vi "Data Channel.vi"(8 "error in (no error)":errorcluster, 11 "Node Ptr":T6 format="%.0x") -> (0 "error out":errorcluster)   [LabVIEW 2018, in "Instrument Addon System Explorer.lvlib"]
uses:
  Instrument Addon System Explorer.lvlib
  <vilib>/NI Veristand/Custom Device API/Custom Device Item Ref.ctl
  Addon Shared/Types/Protocol Data Type.ctl
  Addon Shared/Types/Data Channel Type.ctl
  Addon Shared/Types/Type Cast Type.ctl
  Addon Shared/Types/Endian.ctl
  Addon Shared/Types/FG Control.ctl
  <vilib>/NI Veristand/Custom Device API/Custom Device Channel.ctl
  <vilib>/NI Veristand/Custom Device API/Custom Device Channel Type.ctl
  Addon Shared/SubVIs/Constants.vi
  <vilib>/NI Veristand/Custom Device API/NI VeriStand - Get Item Property.vi
  <vilib>/NI Veristand/Custom Device API/Get Item Property (U32).vi
  <vilib>/NI Veristand/Custom Device API/Get Item Property (String).vi
  <vilib>/NI Veristand/Custom Device API/Get Item Property (String Array).vi
  <vilib>/NI Veristand/Custom Device API/NI VeriStand - Set Item Property.vi
  <vilib>/NI Veristand/Custom Device API/Set Item Property (U32).vi
  <vilib>/NI Veristand/Custom Device API/Set Item Property (String).vi
  <vilib>/NI Veristand/Custom Device API/Set Item Property (String Array).vi
  <vilib>/NI Veristand/Custom Device API/NI VeriStand - Set Custom Device Channel Value Table.vi
  <vilib>/NI Veristand/Custom Device API/Custom Device API.lvlib
  Addon Shared/Instrument Addon Shared.lvlib
panel:
  in  "Delimiter":string=","
  in  "Reset":bool
  in  "Create":bool
  in  "Elements":u32
  in  "Units":string
  in  "Default Value":dbl
  in  "SHDocVw.IWebBrowser":refnum<k7>(container)
  out "Channel Type (Tab)":T1(tab)
  in  "Test Value":dbl
  in  "Format String":string="%.3g"
  out "Validated String":string
  in  "Expected String":string caption="Expected String (case sensitive)"
  in  "Endian":T2=enum."Little"
  in  "Type":T3
  in  "Enumerated List":i32(listbox)
  in  "Add":bool
  in  "Remove":bool
  in  "Channel Type":T4
  out "Data Type":T5
  in  "Header":cluster{"Section Name":string}={"Section Name"="Data Settings"}
  in  "Description":string
  in  "Name":string
  in  "Header 2":cluster{"Section Name":string}={"Section Name"="Data Format Settings"}
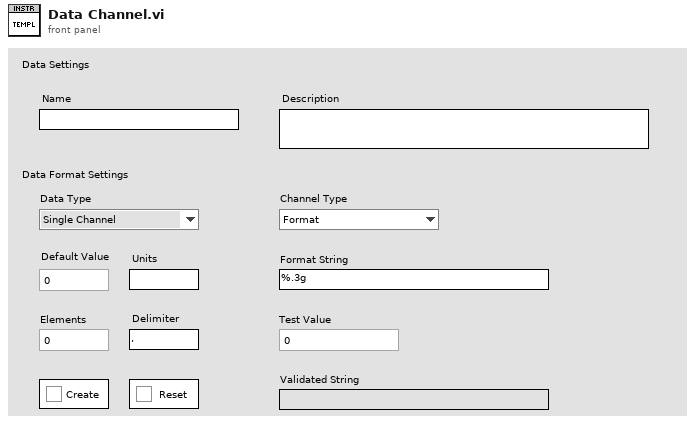
[diagram p1: front panel]
types:
  T1 = enum32{"Format", "Comparison", "Type Cast", "List"}
  T2 = typedef "Instrument Addon Shared.lvlib/Endian.ctl" = enum16{"Native", "Little", "Big"}
  T3 = typedef "Instrument Addon Shared.lvlib/Type Cast Type.ctl" = enum16{"DBL", "SGL", "U64", "U32", "U16", "U8", "I64", "I32", "I16", "I8"}
  T4 = typedef "Instrument Addon Shared.lvlib/Data Channel Type.ctl" = enum16{"Format", "Comparison", "Type Cast", "Enumerated List"}
  T5 = typedef "Instrument Addon Shared.lvlib/Protocol Data Type.ctl" = enum16{"Single Channel", "Array"}
  T6 = typedef "Custom Device API.lvlib/Custom Device Item Ref.ctl" = u64
  T7 = typedef "Instrument Addon Shared.lvlib/FG Control.ctl" = enum16{"Get", "Set"}
  T8 = typedef "Custom Device API.lvlib/Custom Device Item Info.ctl" = cluster{"Name":string, "Is Channel":bool, "GUID":string, "Is Waveform":bool}
  T9 = typedef "Instrument Addon Shared.lvlib/Data Parameters.ctl" = cluster{"Data Type":T5, "Channel Type":T4, "Format String":string, "Expected String":string, "Type":T3, "List":string[], "Delimiter":string, "Endian":T2}
  T10 = typedef "Custom Device API.lvlib/Custom Device Channel.ctl" = cluster{"Type":T11, "Units":string, "Default Value":dbl, "Faultable":bool, "Scalable":bool}
  T11 = typedef "Custom Device API.lvlib/Custom Device Channel Type.ctl" = enum16{"Input", "Output"}
  T12 = typedef "Custom Device API.lvlib/Custom Device Commands.ctl" = enum16{"Default", "Item renamed", "Shutdown", "Dynamic button pressed"}
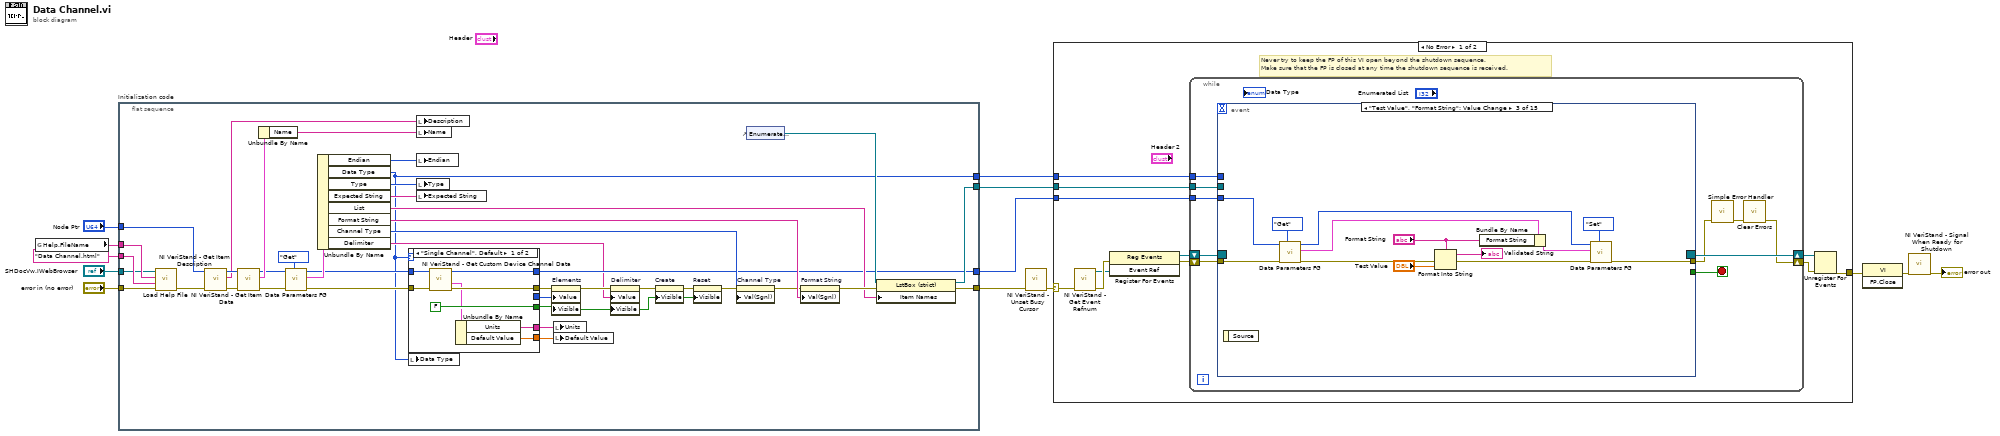
[diagram p0: block diagram]
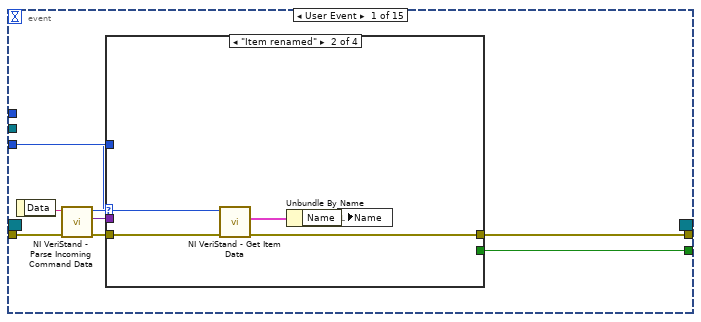
[diagram p2: hidden frame]
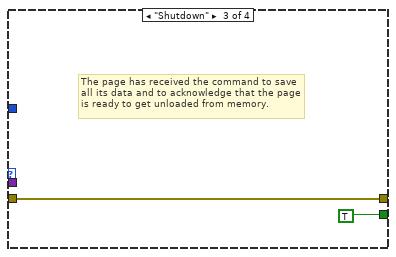
[diagram p4: hidden frame]
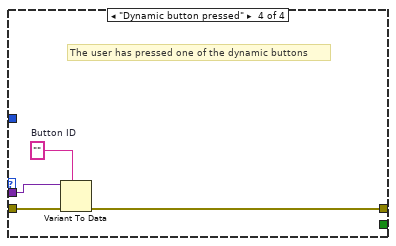
[diagram p5: hidden frame]
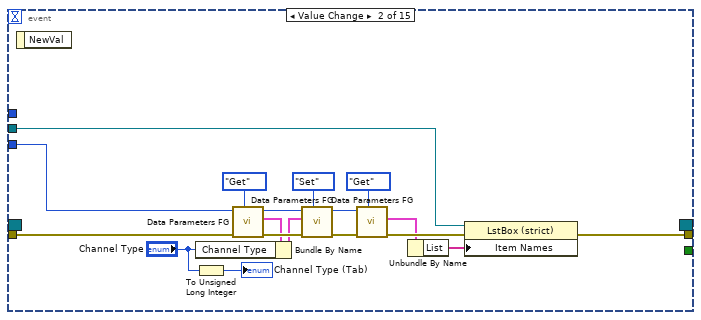
[diagram p6: hidden frame]
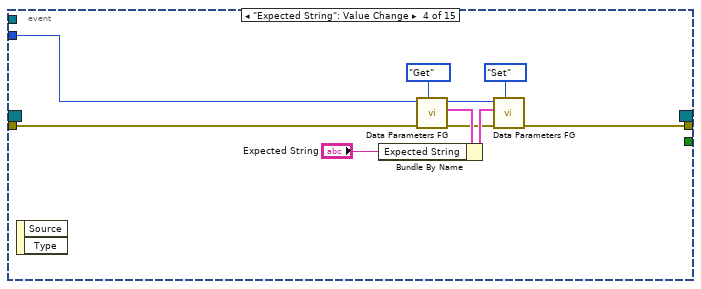
[diagram p7: hidden frame]
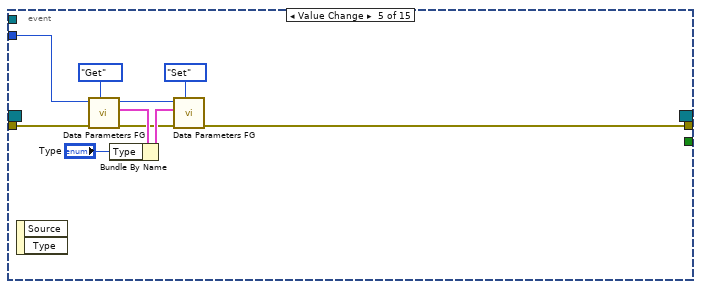
[diagram p8: hidden frame]
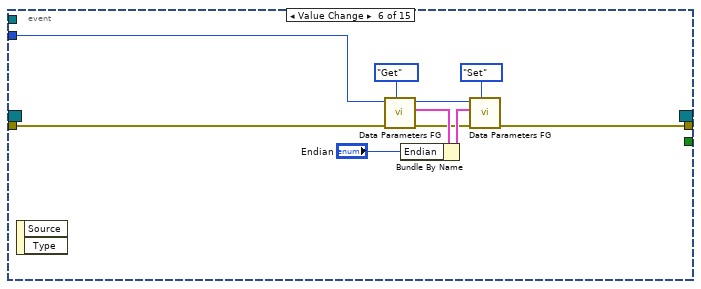
[diagram p9: hidden frame]
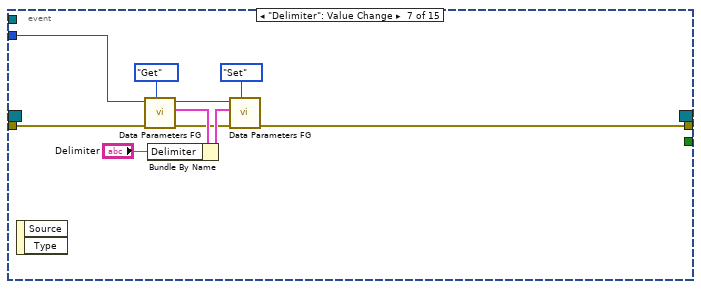
[diagram p10: hidden frame]
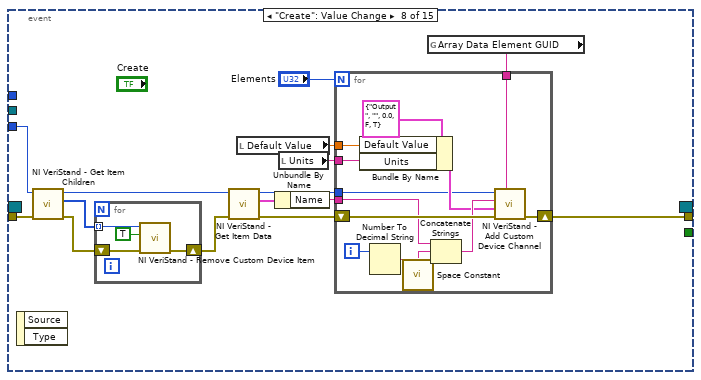
[diagram p11: hidden frame]
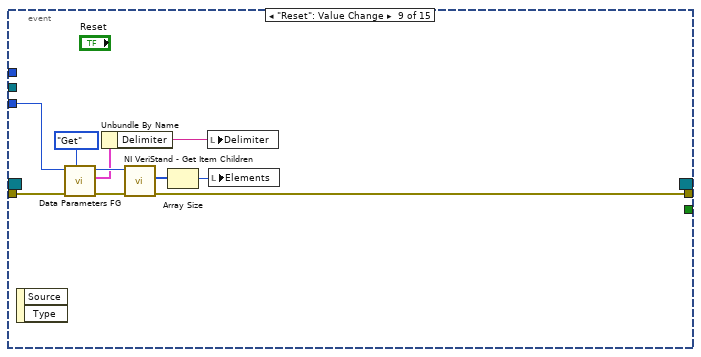
[diagram p12: hidden frame]
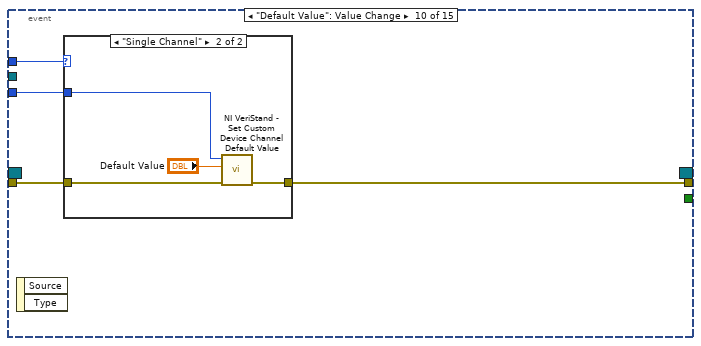
[diagram p13: hidden frame]
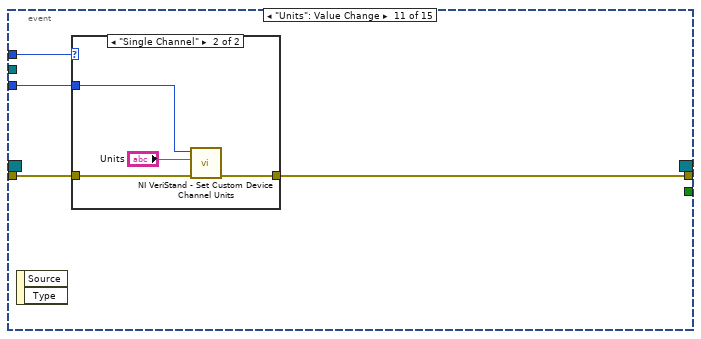
[diagram p15: hidden frame]
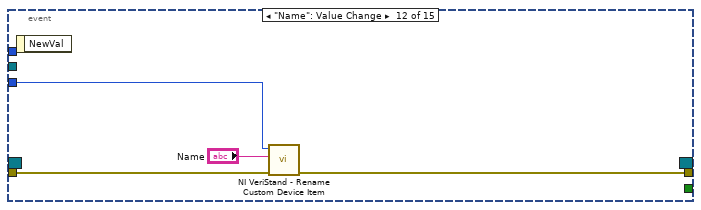
[diagram p17: hidden frame]
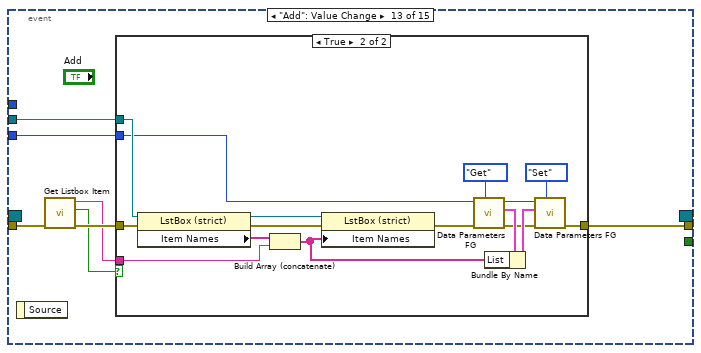
[diagram p18: hidden frame]
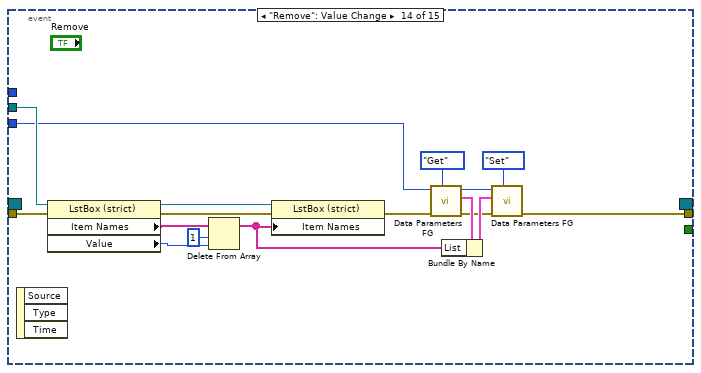
[diagram p20: hidden frame]
diagram:
  n1 = global read "Constants.vi" "Help.FileName"() -> (w1:string)
  n2 = flat-sequence "Initialization code" {
    tunnel: "error in (no error)" -> [w47]
    tunnel: "Node Ptr" -> [w52]
    tunnel: [w34] -> w9
    tunnel: [w26] -> w6
    tunnel: w1 -> [w45]
    tunnel: "Data Channel.html" ("HTML File") -> [w44]
    tunnel: "SHDocVw.IWebBrowser" -> [w43]
    tunnel: [w31] -> w3
    tunnel: [w16] -> w2
    frame #0 {
      n3 = call "Load Help File.vi"("error in (no error)"=w47, "HTML File"=w44, "Main CHM File"=w45, "SHDocVw.IWebBrowser2"=w43) -> ("error out"=w46:errorcluster)  [unwired: 7 in]
      n4 = call <vilib>:"NI VeriStand - Get Item Description.vi"("error in (no error)"=w46, "Item Ref in"=w52) -> ("error out"=w50:errorcluster, "Description"=w51:string, "Item Ref out"=w53:T6)  [unwired: 7 out]
      n5 = call <vilib>:"NI VeriStand - Get Item Data.vi"("error in (no error)"=w50, "Item Ref in"=w53) -> ("error out"=w30:errorcluster, "Item Info"=w49:T8, "Item Ref out"=w29:T6)  [unwired: 7 out]
      n6 = Unbundle By Name(w49) -> ("Name"=w48:string)
      n7 = call "Data Parameters FG.vi"("Action"=FG_Control."Get", "error in (no error)"=w30, "Item Ref in"=w29) -> ("error out"=w28:errorcluster, "Data Parameters"=w41:T9, "Item Ref out"=w27:T6)  [unwired: 6 in]
      n8 = Unbundle By Name(w41) -> ("Endian"=w15:T2, "Data Type"=w16:T5, "Type"=w36:T3, "Expected String"=w37:string, "List"=w32:string[], "Format String"=w40:string, "Channel Type"=w39:T4, "Delimiter"=w17:string)
      n9 = case shown="\"Single Channel\", Default" w16 {
        tunnel: [FALSE TRUE] -> w14
        tunnel: w28 -> [w60 w65]
        tunnel: w27 -> [w59 w69]
        tunnel: [w58 w64] -> w19
        tunnel: [w57 w66] -> w26
        tunnel: [w55 ""] -> w25
        tunnel: [w54 0.0 ("Default Value")] -> w24
        tunnel: [_ w62] -> w18
        frame "Single Channel", Default {
          n10 = call <vilib>:"NI VeriStand - Get Custom Device Channel Data.vi"("error in (no error)"=w60, "Channel Ref in"=w59) -> ("error out"=w58:errorcluster, "Channel"=w56:T10, "Channel Ref out"=w57:T6)  [unwired: 4 in, 3 out]
          n11 = Unbundle By Name(w56) -> ("Units"=w55:string, "Default Value"=w54:dbl)
        }
        frame "Array" {
          n12 = call <vilib>:"NI VeriStand - Get Item Children.vi"("error in (no error)"=w65, "Item Ref in"=w69) -> ("error out"=w64:errorcluster, "Child Refs"=w63:T6[], "Item Ref out"=w66:T6)  [unwired: 6 in, 1 out]
          n13 = Array Size(array=w63) -> (size(s)=w62:i32)
        }
      }
      n14 = local write "Data Type"(w16) -> ()
      n15 = local write "Description"(w51) -> ()
      n16 = local write "Name"(w48) -> ()
      n17 = local write "Endian"(w15) -> ()
      n18 = local write "Type"(w36) -> ()
      n19 = local write "Expected String"(w37) -> ()
      n20 = property on="Elements" class="DigNum (strict)"(error in=w19, "Value"=w18, "Visible"=w14) -> (error out=w23:errorcluster)  [unwired: 1 in, 1 out]
      n21 = local write "Units"(w25) -> ()
      n22 = local write "Default Value"(w24) -> ()
      n23 = property on="Delimiter" class="Str"(error in=w23, "Value"=w17, "Visible"=w14) -> (error out=w22:errorcluster)  [unwired: 1 in, 1 out]
      n24 = property on="Create" class="Bool"(error in=w22, "Visible"=w14) -> (error out=w21:errorcluster)  [unwired: 1 in, 1 out]
      n25 = property on="Reset" class="Bool"(error in=w21, "Visible"=w14) -> (error out=w20:errorcluster)  [unwired: 1 in, 1 out]
      n26 = property on="Channel Type" class="Enum (strict)"(error in=w20, "Val(Sgnl)"=w39) -> (error out=w38:errorcluster)  [unwired: 1 in, 1 out]
      n27 = control-ref of="Enumerated List"() -> (w33:refnum<vi>)
      n28 = property on="Format String" class="Str"(error in=w38, "Val(Sgnl)"=w40) -> (error out=w35:errorcluster)  [unwired: 1 in, 1 out]
      n29 = property class="LstBox (strict)"(reference=w33, error in=w35, "Item Names"=w32) -> (reference out=w31:refnum<vi>, error out=w34:errorcluster)
    }
  }
  n30 = call <vilib>:"NI VeriStand - Unset Busy Cursor.vi"("error in (no error)"=w9) -> ("error out"=w8:errorcluster)  [unwired: 10 out]
  n31 = case shown="No Error" w8 {
    selector: w8 -> [w73 w294]
    tunnel: [w78 w292] -> w13
    tunnel: w6 -> [w74 _]
    tunnel: w3 -> [w72 _]
    tunnel: w2 -> [w71 _]
    frame No Error {
      # "Never try to keep the FP of this VI open beyond the shutdown sequence.\nMake sure that the FP is closed at any time the shutdown sequence is received."
      n32 = call <vilib>:"NI VeriStand - Get Event Refnum.vi"("error in (no error)"=w73) -> ("error out"=w81:errorcluster, "Event Ref"=w77:refnum<user-event>)  [unwired: 9 out]
      n33 = register-events(error in=w81, w77) -> (reference out=w75:refnum<event-registration>, error out=w76:errorcluster)  [unwired: 1 in]
      n34 = while {
        tunnel: w74 -> [w87]
        shift-right: [w84] -> w79
        shift-left: w76 -> [w90]
        shift-right: [w91] -> w80
        shift-left: w75 -> [w89]
        tunnel: w72 -> [w83]
        tunnel: w71 -> [w82]
        stop <- w88 stop-if-true
        n35 = event shown="[2] \"Test Value\", \"Format String\": Value Change" {
          selector: w89 -> [_ _ _ _ _ _ _ _ _ _ _ _ _ _ _]
          dyn-events: [_ _ _ _ _ _ _ _ _ _ _ _ _ _ _] -> w91
          timeout: _ -> [_ _ _ _ _ _ _ _ _ _ _ _ _ _ _]
          tunnel: w90 -> [w99 w123 w140 w150 w160 w170 w180 w184 w222 w228 w237 w246 w248 w273 w290]
          tunnel: [w95 _ _ _ _ _ _ _ _ _ _ _ _ _ _] -> w88
          tunnel: [w94 w112 w139 w149 w153 w169 w179 w186 w215 w227 w236 w245 w247 w274 w289] -> w86
          tunnel: w87 -> [w93 w121 w138 w148 w159 w168 w178 w183 w220 w226 w235 w244 w250 w271 w291]
          tunnel: w83 -> [_ w114 _ _ _ _ _ _ _ _ _ _ w249 w272 _]
          tunnel: w82 -> [_ _ _ _ _ _ _ _ _ w225 w234 _ _ _ _]
          event User Event {
            n36 = event-data() -> ("Data"=w98:string)  [unwired: 1 out]
            n37 = call <vilib>:"NI VeriStand - Parse Incoming Command Data.vi"("error in (no error)"=w99, "Incoming data"=w98) -> ("error out"=w97:errorcluster, "Outgoing data"=w92:variant, "Action"=w96:T12)  [unwired: 7 out]
            n38 = case shown="\"Item renamed\"" w96 {
              tunnel: w97 -> [w100 w105 w106 w111]
              tunnel: [_ _ TRUE _] -> w95
              tunnel: [w100 w102 w106 w108] -> w94
              tunnel: w93 -> [_ w104 _ _]
              tunnel: w92 -> [_ _ _ w110]
              frame "Default", Default {
              }
              frame "Item renamed" {
                n39 = call <vilib>:"NI VeriStand - Get Item Data.vi"("error in (no error)"=w105, "Item Ref in"=w104) -> ("error out"=w102:errorcluster, "Item Info"=w103:T8)  [unwired: 8 out]
                n40 = Unbundle By Name(w103) -> ("Name"=w101:string)
                n41 = local write "Name"(w101) -> ()
              }
              frame "Shutdown" {
                # "The page has received the command to save all its data and to acknowledge that the page is ready to get unloaded from memory."
              }
              frame "Dynamic button pressed" {
                w109 = ""  # Button ID
                # "The user has pressed one of the dynamic buttons"
                n42 = Variant To Data(error in=w111, type=w109, Variant=w110) -> (error out=w108:errorcluster)  [unwired: 1 out]
              }
            }
          }
          event Value Change {
            n43 = event-data() -> ()  [unwired: 2 out]
            n44 = To Unsigned Long Integer(number="Channel Type") -> (unsigned 32bit integer=→"Channel Type (Tab)":u32)
            n45 = call "Data Parameters FG.vi"("Action"=FG_Control."Get", "error in (no error)"=w123, "Item Ref in"=w121) -> ("error out"=w129:errorcluster, "Data Parameters"=w125:T9, "Item Ref out"=w127:T6)  [unwired: 6 in]
            n46 = Bundle By Name(cluster=w125, "Channel Type"="Channel Type") -> (w126:T9)
            n47 = call "Data Parameters FG.vi"("Action"=FG_Control."Set", "error in (no error)"=w129, "Data Parameters"=w126, "Item Ref in"=w127) -> ("error out"=w116:errorcluster, "Item Ref out"=w115:T6)  [unwired: 5 in, 1 out]
            n48 = call "Data Parameters FG.vi"("Action"=FG_Control."Get", "error in (no error)"=w116, "Item Ref in"=w115) -> ("error out"=w119:errorcluster, "Data Parameters"=w118:T9)  [unwired: 6 in, 1 out]
            n49 = Unbundle By Name(w118) -> ("List"=w117:string[])
            n50 = property class="LstBox (strict)"(reference=w114, error in=w119, "Item Names"=w117) -> (error out=w112:errorcluster)  [unwired: 1 out]
          }
          event "Test Value", "Format String": Value Change {
            n51 = event-data() -> ()  [unwired: 2 out]
            n52 = call "Data Parameters FG.vi"("Action"=FG_Control."Get", "error in (no error)"=w140, "Item Ref in"=w138) -> ("error out"=w134:errorcluster, "Data Parameters"=w130:T9, "Item Ref out"=w131:T6)  [unwired: 6 in]
            n53 = Format Into String(format string="Format String", error in=w134, "Test Value") -> (resulting string=→"Validated String":string, error out=w133:errorcluster)  [unwired: 1 in]
            n54 = Bundle By Name(cluster=w130, "Format String"="Format String") -> (w132:T9)
            n55 = call "Data Parameters FG.vi"("Action"=FG_Control."Set", "error in (no error)"=w133, "Data Parameters"=w132, "Item Ref in"=w131) -> ("error out"=w139:errorcluster)  [unwired: 5 in, 2 out]
          }
          event "Expected String": Value Change {
            n56 = event-data() -> ()  [unwired: 3 out]
            n57 = call "Data Parameters FG.vi"("Action"=FG_Control."Get", "error in (no error)"=w150, "Item Ref in"=w148) -> ("error out"=w143:errorcluster, "Data Parameters"=w145:T9, "Item Ref out"=w146:T6)  [unwired: 6 in]
            n58 = Bundle By Name(cluster=w145, "Expected String"="Expected String") -> (w147:T9)
            n59 = call "Data Parameters FG.vi"("Action"=FG_Control."Set", "error in (no error)"=w143, "Data Parameters"=w147, "Item Ref in"=w146) -> ("error out"=w149:errorcluster)  [unwired: 5 in, 2 out]
          }
          event Value Change {
            n60 = event-data() -> ()  [unwired: 3 out]
            n61 = call "Data Parameters FG.vi"("Action"=FG_Control."Get", "error in (no error)"=w160, "Item Ref in"=w159) -> ("error out"=w155:errorcluster, "Data Parameters"=w156:T9, "Item Ref out"=w157:T6)  [unwired: 6 in]
            n62 = Bundle By Name(cluster=w156, "Type"="Type") -> (w158:T9)
            n63 = call "Data Parameters FG.vi"("Action"=FG_Control."Set", "error in (no error)"=w155, "Data Parameters"=w158, "Item Ref in"=w157) -> ("error out"=w153:errorcluster)  [unwired: 5 in, 2 out]
          }
          event Value Change {
            n64 = event-data() -> ()  [unwired: 3 out]
            n65 = call "Data Parameters FG.vi"("Action"=FG_Control."Get", "error in (no error)"=w170, "Item Ref in"=w168) -> ("error out"=w164:errorcluster, "Data Parameters"=w165:T9, "Item Ref out"=w166:T6)  [unwired: 6 in]
            n66 = Bundle By Name(cluster=w165, "Endian"="Endian") -> (w167:T9)
            n67 = call "Data Parameters FG.vi"("Action"=FG_Control."Set", "error in (no error)"=w164, "Data Parameters"=w167, "Item Ref in"=w166) -> ("error out"=w169:errorcluster)  [unwired: 5 in, 2 out]
          }
          event "Delimiter": Value Change {
            n68 = event-data() -> ()  [unwired: 3 out]
            n69 = call "Data Parameters FG.vi"("Action"=FG_Control."Get", "error in (no error)"=w180, "Item Ref in"=w178) -> ("error out"=w174:errorcluster, "Data Parameters"=w175:T9, "Item Ref out"=w176:T6)  [unwired: 6 in]
            n70 = Bundle By Name(cluster=w175, "Delimiter"="Delimiter") -> (w177:T9)
            n71 = call "Data Parameters FG.vi"("Action"=FG_Control."Set", "error in (no error)"=w174, "Data Parameters"=w177, "Item Ref in"=w176) -> ("error out"=w179:errorcluster)  [unwired: 5 in, 2 out]
          }
          event "Create": Value Change {
            n72 = event-data() -> ()  [unwired: 3 out]
            n73 = call <vilib>:"NI VeriStand - Get Item Children.vi"("error in (no error)"=w184, "Item Ref in"=w183) -> ("error out"=w197:errorcluster, "Child Refs"=w196:T6[], "Item Ref out"=w194:T6)  [unwired: 6 in, 1 out]
            n74 = for {
              shift-right: [w200] -> w195
              shift-left: w197 -> [w198]
              tunnel: w196 -> [w199] mode=indexing
              n75 = call <vilib>:"NI VeriStand - Remove Custom Device Item.vi"("error in (no error)"=w198, "Force Delete (F)"=TRUE, "Item Ref in"=w199) -> ("error out"=w200:errorcluster)  [unwired: 7 in, 1 out]
            }
            n76 = call <vilib>:"NI VeriStand - Get Item Data.vi"("error in (no error)"=w195, "Item Ref in"=w194) -> ("error out"=w188:errorcluster, "Item Info"=w187:T8, "Item Ref out"=w193:T6)  [unwired: 7 out]
            n77 = local read "Default Value"() -> (w191:dbl)
            n78 = Unbundle By Name(w187) -> ("Name"=w189:string)
            n79 = local read "Units"() -> (w190:string)
            n80 = global read "Constants.vi" "Array Data Element GUID"() -> (w192:string)
            n81 = for {
              N: "Elements" -> [_]
              shift-right: [w213] -> w186
              shift-left: w188 -> [w214]
              tunnel: w189 -> [w211]
              tunnel: w190 -> [w205]
              tunnel: w191 -> [w204]
              tunnel: w192 -> [w203]
              tunnel: w193 -> [w202]
              i -> [w212]
              n82 = Bundle By Name(cluster=T10 {"Type"=enum."Output", "Units"="", "Default Value"=0.0, "Faultable"=FALSE, "Scalable"=TRUE} ("Channel"), "Default Value"=w204, "Units"=w205) -> (w206:T10)
              n83 = Number To Decimal String(number=w212) -> (decimal integer string=w210:string)  [unwired: 1 in]
              n84 = call <vilib>:"Space Constant.vi"() -> ("String"=w209:string)
              n85 = Concatenate Strings(w211, w209, w210) -> (w208:string)
              n86 = call <vilib>:"NI VeriStand - Add Custom Device Channel.vi"("GUID (Default Channel)"=w203, "error in (no error)"=w214, "Channel"=w206, "Channel Name"=w208, "Parent Ref in"=w202) -> ("error out"=w213:errorcluster)  [unwired: 3 in, 3 out]
            }
          }
          event "Reset": Value Change {
            n87 = event-data() -> ()  [unwired: 3 out]
            n88 = call "Data Parameters FG.vi"("Action"=FG_Control."Get", "error in (no error)"=w222, "Item Ref in"=w220) -> ("error out"=w221:errorcluster, "Data Parameters"=w218:T9, "Item Ref out"=w219:T6)  [unwired: 6 in]
            n89 = Unbundle By Name(w218) -> ("Delimiter"=w217:string)
            n90 = call <vilib>:"NI VeriStand - Get Item Children.vi"("error in (no error)"=w221, "Item Ref in"=w219) -> ("error out"=w215:errorcluster, "Child Refs"=w224:T6[])  [unwired: 6 in, 2 out]
            n91 = Array Size(array=w224) -> (size(s)=w216:i32)
            n92 = local write "Delimiter"(w217) -> ()
            n93 = local write "Elements"(w216) -> ()
          }
          event "Default Value": Value Change {
            n94 = event-data() -> ()  [unwired: 3 out]
            n95 = case shown="\"Single Channel\"" w225 {
              tunnel: w228 -> [w229 w233]
              tunnel: [w229 w232] -> w227
              tunnel: w226 -> [_ w231]
              frame "Array" {
              }
              frame "Single Channel" {
                n96 = call <vilib>:"NI VeriStand - Set Custom Device Channel Default Value.vi"("error in (no error)"=w233, "Default Value"="Default Value", "Channel Ref in"=w231) -> ("error out"=w232:errorcluster)  [unwired: 7 in, 1 out]
              }
            }
          }
          event "Units": Value Change {
            n97 = event-data() -> ()  [unwired: 3 out]
            n98 = case shown="\"Single Channel\"" w234 {
              tunnel: w237 -> [w238 w242]
              tunnel: [w238 w241] -> w236
              tunnel: w235 -> [_ w240]
              frame "Array" {
              }
              frame "Single Channel" {
                n99 = call <vilib>:"NI VeriStand - Set Custom Device Channel Units.vi"("error in (no error)"=w242, "Units"="Units", "Channel Ref in"=w240) -> ("error out"=w241:errorcluster)  [unwired: 7 in, 1 out]
              }
            }
          }
          event "Name": Value Change {
            n100 = event-data() -> ()  [unwired: 2 out]
            n101 = call <vilib>:"NI VeriStand - Rename Custom Device Item.vi"("error in (no error)"=w246, "New Name"="Name", "Item Ref in"=w244) -> ("error out"=w245:errorcluster)  [unwired: 1 in, 7 out]
          }
          event "Add": Value Change {
            n102 = event-data() -> ()  [unwired: 2 out]
            n103 = call "Get Listbox Item.vi"("error in (no error)"=w248) -> ("error out"=w253:errorcluster, "OK?"=w252:bool, "Item out"=w251:string)  [unwired: 8 in]
            n104 = case shown="True" w252 {
              tunnel: w249 -> [_ w270]
              tunnel: w253 -> [w254 w269]
              tunnel: w251 -> [_ w265]
              tunnel: [w254 w256] -> w247
              tunnel: w250 -> [_ w258]
              frame False {
              }
              frame True {
                n105 = property class="LstBox (strict)"(reference=w270, error in=w269) -> (reference out=w268:refnum<vi>, error out=w267:errorcluster, "Item Names"=w266:string[])
                n106 = Build Array (concatenate)(w266, w265) -> (w255:string[])
                n107 = property class="LstBox (strict)"(reference=w268, error in=w267, "Item Names"=w255) -> (error out=w257:errorcluster)  [unwired: 1 out]
                n108 = call "Data Parameters FG.vi"("Action"=FG_Control."Get", "error in (no error)"=w257, "Item Ref in"=w258) -> ("error out"=w259:errorcluster, "Data Parameters"=w263:T9, "Item Ref out"=w261:T6)  [unwired: 6 in]
                n109 = Bundle By Name(cluster=w263, "List"=w255) -> (w262:T9)
                n110 = call "Data Parameters FG.vi"("Action"=FG_Control."Set", "error in (no error)"=w259, "Data Parameters"=w262, "Item Ref in"=w261) -> ("error out"=w256:errorcluster)  [unwired: 5 in, 2 out]
              }
            }
          }
          event "Remove": Value Change {
            n111 = event-data() -> ()  [unwired: 4 out]
            n112 = property class="LstBox (strict)"(reference=w272, error in=w273) -> (reference out=w283:refnum<vi>, error out=w284:errorcluster, "Item Names"=w285:string[], "Value"=w286:i32)
            n113 = Delete From Array(array=w285, length=1, index=w286) -> (array with subset deleted=w275:string[])  [unwired: 1 out]
            n114 = property class="LstBox (strict)"(reference=w283, error in=w284, "Item Names"=w275) -> (error out=w276:errorcluster)  [unwired: 1 out]
            n115 = call "Data Parameters FG.vi"("Action"=FG_Control."Get", "error in (no error)"=w276, "Item Ref in"=w271) -> ("error out"=w277:errorcluster, "Data Parameters"=w281:T9, "Item Ref out"=w279:T6)  [unwired: 6 in]
            n116 = Bundle By Name(cluster=w281, "List"=w275) -> (w280:T9)
            n117 = call "Data Parameters FG.vi"("Action"=FG_Control."Set", "error in (no error)"=w277, "Data Parameters"=w280, "Item Ref in"=w279) -> ("error out"=w274:errorcluster)  [unwired: 5 in, 2 out]
          }
          event "Description": Value Change {
            n118 = event-data() -> ()  [unwired: 2 out]
            n119 = call <vilib>:"NI VeriStand - Set Item Description.vi"("error in (no error)"=w290, "Description"="Description", "Item Ref in"=w291) -> ("error out"=w289:errorcluster)  [unwired: 8 out]
          }
        }
        n120 = call <vilib>:"Simple Error Handler.vi"("error in (no error)"=w86) -> ("error out"=w85:errorcluster)  [unwired: 1 in, 7 out]
        n121 = call <vilib>:"Clear Errors.vi"("error in (no error)"=w85) -> ("error out"=w84:errorcluster)  [unwired: 1 in, 5 out]
      }
      n122 = Unregister For Events(event registration refnum=w80, error in=w79) -> (error out=w78:errorcluster)
    }
    frame Error {
      n123 = call <vilib>:"Simple Error Handler.vi"("error in (no error)"=w294) -> ("error out"=w293:errorcluster)  [unwired: 1 in, 7 out]
      n124 = call <vilib>:"Clear Errors.vi"("error in (no error)"=w293) -> ("error out"=w292:errorcluster)  [unwired: 1 in, 5 out]
    }
  }
  n125 = invoke class="VI" method="FP.Close"(error in=w13) -> (error out=w12:errorcluster)  [unwired: 2 in, 2 out]
  n126 = call <vilib>:"NI VeriStand - Signal When Ready for Shutdown.vi"("error in (no error)"=w12) -> ("error out"=→"error out":errorcluster)  [unwired: 10 out]
